vi "Clear Graph.vi"(8 "error in (no error)":errorcluster, 11 "Live Graph Plotter in":refnum<class "Live Graph Plotter.lvclass">) -> (0 "error out":errorcluster, 3 "Live Graph Plotter out":refnum<class "Live Graph Plotter.lvclass">)   [LabVIEW 2025, in "Live Graph Plotter.lvclass"]
uses:
  Live Graph Plotter.lvclass
  Live Graph Plotter.lvclass/Live Graph Plotter.ctl
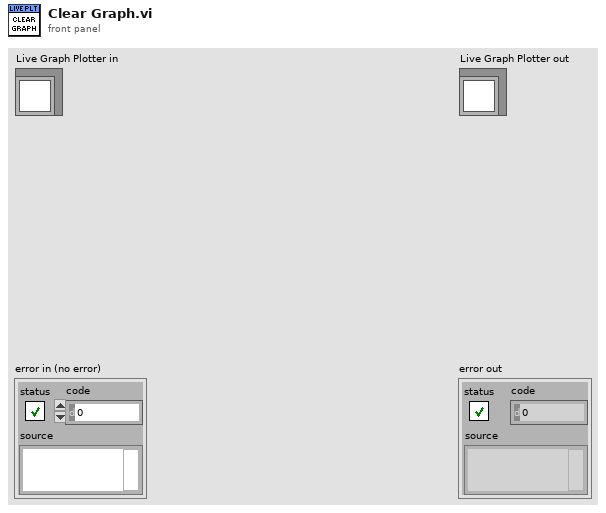
[diagram p1: front panel]
types:
  T1 = cluster{"relativeInitialX":dbl, "xIncrement":dbl, "wfm":dbl[]}[]
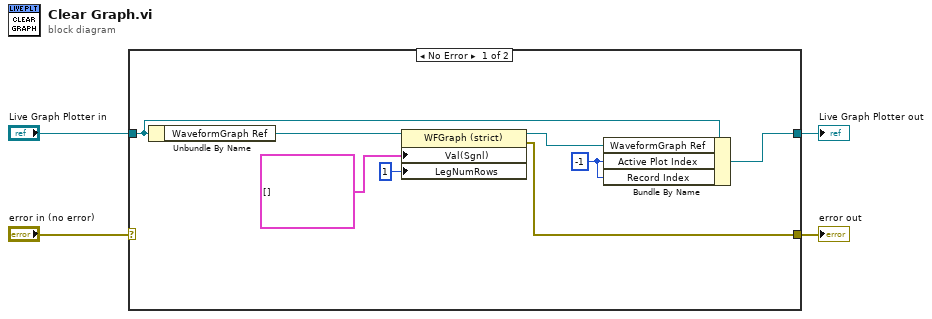
[diagram p0: block diagram]
diagram:
  n1 = case shown="No Error" "error in (no error)" {
    selector: "error in (no error)" -> [_ w14]
    tunnel: [w8 w14] -> w3
    tunnel: [w9 w13] -> w1
    tunnel: "Live Graph Plotter in" -> [w12 w13]
    frame No Error {
      w6 = -1 ("Active Plot Index")
      n2 = Unbundle By Name(w12) -> ("WaveformGraph Ref"=w11:refnum<vi>)
      n3 = property class="WFGraph (strict)"(reference=w11, "Val(Sgnl)"=T1 [] ("Value (Signaling)"), "LegNumRows"=u32 1 ("Legend:Number of Rows")) -> (reference out=w7:refnum<vi>, error out=w8:errorcluster)  [unwired: 1 in]
      n4 = Bundle By Name(cluster=w12, "WaveformGraph Ref"=w7, "Active Plot Index"=w6, "Record Index"=w6) -> (w9:refnum<class "Live Graph Plotter.lvclass">)
    }
    frame Error {
    }
  }
  "error out" <- w3
  "Live Graph Plotter out" <- w1
